vi "OscillationTracker35Hz.vi"(0 "input data":i16) -> (4 "Amplitude":i16, 6 "Ascending":bool, 8 "Descending":bool, 10 "Peak":bool, 15 "Trough":bool)   [LabVIEW 2019]
uses:
  <vilib>/rvi/Analysis/measure/butterworth/XNode/niFpgaButterworthFilter.xnode
  <vilib>/rvi/Analysis/common/FxpNativeNode/niFpgaFxpNative.xnode
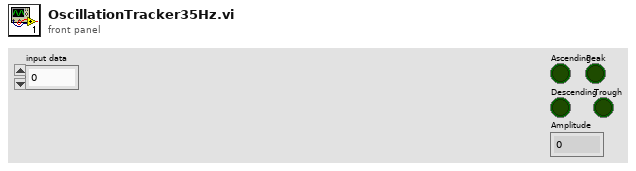
[diagram p1: front panel]
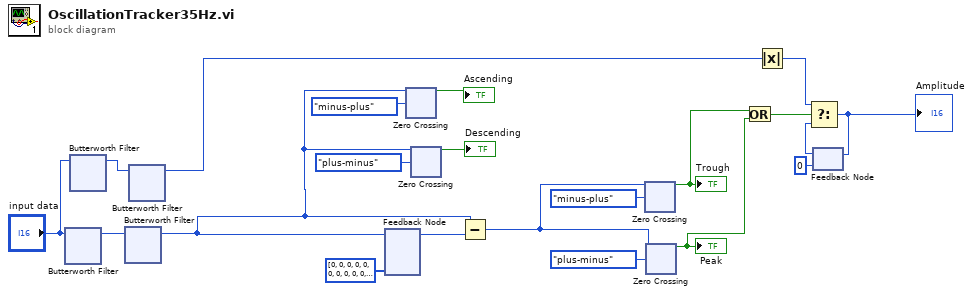
[diagram p0: block diagram]
diagram:
  n1 = xnode "Butterworth Filter"("input data"="input data") -> ("output data"=w8:i16)  [unwired: 2 in]
  n2 = xnode "Butterworth Filter"("input data"="input data") -> ("output data"=w1:i16)  [unwired: 2 in]
  n3 = xnode "Butterworth Filter"("input data"=w8) -> ("output data"=w7:i16)  [unwired: 2 in]
  n4 = xnode "Butterworth Filter"("input data"=w1) -> ("output data"=w6:i16)  [unwired: 2 in]
  n5 = feedback #1(i16[] [0, 0, 0, 0, 0, 0, 0, 0, 0, 0, 0, 0, 0, 0, 0, 0, 0, 0, 0, 0, 0, 0, 0, 0, 0, 0, 0, 0, 0, 0, 0, 0, 0, 0, 0, 0, 0, 0, 0, 0, 0, 0, 0, 0, 0, 0, 0, 0, 0, 0]) -> (w16:i16)
  n6 = feedback-in #1(w7) -> ()
  n7 = xnode ("Zero Crossing")("direction"=enum8{"either", "minus-plus", "plus-minus"}."minus-plus", "input"=w7) -> ("crossing"=→"Ascending":bool)  [unwired: 1 in]
  n8 = xnode ("Zero Crossing")("direction"=enum8{"either", "minus-plus", "plus-minus"}."plus-minus", "input"=w7) -> ("crossing"=→"Descending":bool)  [unwired: 1 in]
  n9 = Subtract(x=w7, y=w16) -> (x-y=w18:i16)
  n10 = xnode ("Zero Crossing")("direction"=enum8{"either", "minus-plus", "plus-minus"}."minus-plus", "input"=w18) -> ("crossing"=w5:bool)  [unwired: 1 in]
  "Trough" <- w5
  n11 = xnode ("Zero Crossing")("direction"=enum8{"either", "minus-plus", "plus-minus"}."plus-minus", "input"=w18) -> ("crossing"=w4:bool)  [unwired: 1 in]
  "Peak" <- w4
  n12 = Or(x=w5, y=w4) -> (x .or. y?=w13:bool)
  n13 = Absolute Value(x=w6) -> (abs(x)=w12:i16)
  n14 = feedback #2(i16 0) -> (w11:i16)
  n15 = Select(t=w12, s=w13, f=w11) -> (s? t:f=w10:i16)
  "Amplitude" <- w10
  n16 = feedback-in #2(w10) -> ()
